vi "da Eq.vi"(0 "Plane Lat":dbl, 1 "Plane Lon":dbl, 2 "Plane Height (ft)":dbl, 3 "Plane Roll":dbl, 4 "Plane Pitch":dbl, 5 "Plane Heading":dbl, 6 "Displayed Image:Size:All Elements":cluster{"Width":u32, "Height":u32}, 7 "Last Mouse Position:All Elements":cluster{"X":i32, "Y":i32}) -> (16 "Latitude":dbl, 17 "Longitude":dbl)   [LabVIEW 2014]
panel:
  in  "Horizontal View Angle":dbl=74.0
  in  "Verticle View Angle":dbl=60.0
  # "AXIS 207MW has a horizontal view angle of 74 deg\nand a verticle view angle of 60 deg"
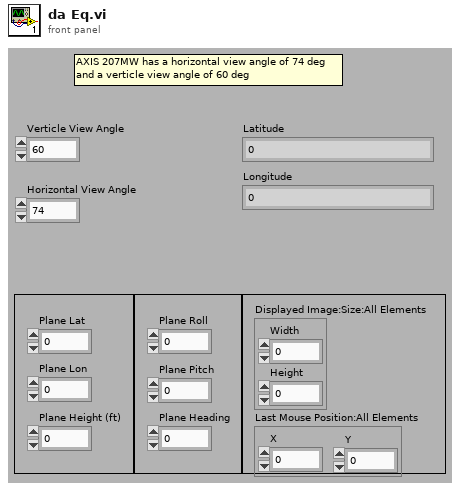
[diagram p1: front panel]
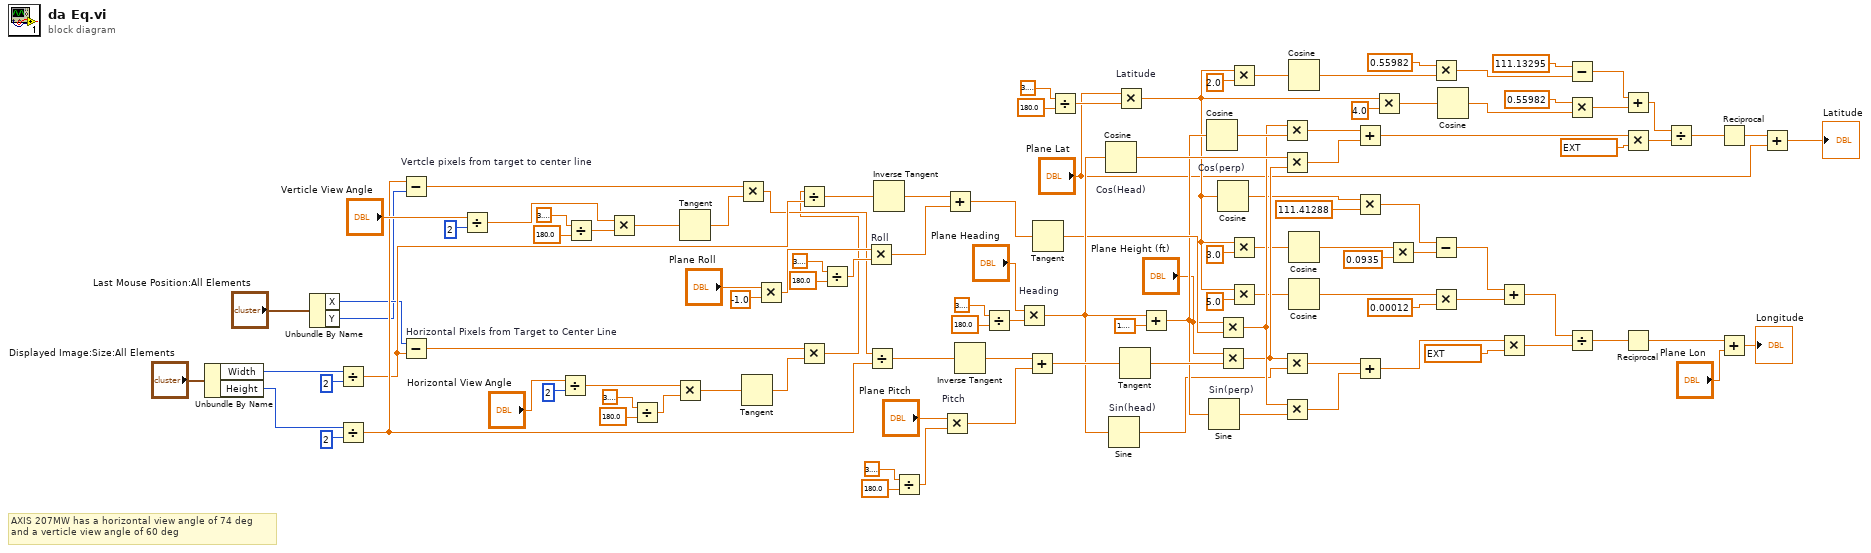
[diagram p0: block diagram]
diagram:
  # "AXIS 207MW has a horizontal view angle of 74 deg\nand a verticle view angle of 60 deg"
  n1 = Unbundle By Name("Displayed Image:Size:All Elements") -> ("Width"=w53:u32, "Height"=w52:u32)
  n2 = Unbundle By Name("Last Mouse Position:All Elements") -> ("X"=w4:i32, "Y"=w3:i32)
  n3 = Divide(x=w53, y=u32 2) -> (x/y=w82:dbl)
  n4 = Divide(x=w52, y=u32 2) -> (x/y=w108:dbl)
  n5 = Subtract "Vertcle pixels from target to center line"(x=w108, y=w3) -> (x-y=w109:dbl)
  n6 = Subtract "Horizontal Pixels from Target to Center Line"(x=w4, y=w82) -> (x-y=w91:dbl)
  n7 = Divide(x="Verticle View Angle", y=u32 2) -> (x/y=w107:dbl)
  n8 = Divide(x="Horizontal View Angle", y=u32 2) -> (x/y=w87:dbl)
  n9 = Divide(x=3.141592653589793, y=180.0) -> (x/y=w104:dbl)
  n10 = Multiply(x=w107, y=w104) -> (x*y=w103:dbl)
  n11 = Divide(x=3.141592653589793, y=180.0) -> (x/y=w90:dbl)
  n12 = Multiply(x=w87, y=w90) -> (x*y=w84:dbl)
  n13 = Tangent(1:w103) -> (0:w102:dbl)
  n14 = Multiply(x=w109, y=w102) -> (x*y=w2:dbl)
  n15 = Tangent(1:w84) -> (0:w83:dbl)
  n16 = Multiply(x="Plane Roll", y=-1.0) -> (x*y=w6:dbl)
  n17 = Multiply(x=w91, y=w83) -> (x*y=w1:dbl)
  n18 = Divide(x=w1, y=w82) -> (x/y=w81:dbl)
  n19 = Divide(x=3.141592653589793, y=180.0) -> (x/y=w77:dbl)
  n20 = Multiply "Roll"(x=w6, y=w77) -> (x*y=w76:dbl)
  n21 = Divide(x=w2, y=w108) -> (x/y=w101:dbl)
  n22 = Inverse Tangent(1:w81) -> (0:w80:dbl)
  n23 = Divide(x=3.141592653589793, y=180.0) -> (x/y=w99:dbl)
  n24 = Multiply "Pitch"(x="Plane Pitch", y=w99) -> (x*y=w96:dbl)
  n25 = Add(x=w80, y=w76) -> (x+y=w75:dbl)
  n26 = Inverse Tangent(1:w101) -> (0:w100:dbl)
  n27 = Divide(x=3.141592653589793, y=180.0) -> (x/y=w92:dbl)
  n28 = Multiply "Heading"(x="Plane Heading", y=w92) -> (x*y=w51:dbl)
  n29 = Add(x=w100, y=w96) -> (x+y=w95:dbl)
  n30 = Tangent(1:w75) -> (0:w50:dbl)
  n31 = Divide(x=3.141592653589793, y=180.0) -> (x/y=w66:dbl)
  n32 = Cosine "Cos(Head)"(x=w51) -> (cos(x)=w48:dbl)
  n33 = Sine "Sin(head)"(x=w51) -> (sin(x)=w41:dbl)
  n34 = Multiply "Latitude"(x="Plane Lat", y=w66) -> (x*y=w25:dbl)
  n35 = Tangent(1:w95) -> (0:w49:dbl)
  n36 = Add(x=w51, y=1.5707963267948966) -> (x+y=w47:dbl)
  n37 = Cosine "Cos(perp)"(x=w47) -> (cos(x)=w45:dbl)
  n38 = Sine "Sin(perp)"(x=w47) -> (sin(x)=w43:dbl)
  n39 = Cosine(x=w25) -> (cos(x)=w35:dbl)
  n40 = Multiply(x="Plane Height (ft)", y=w50) -> (x*y=w42:dbl)
  n41 = Multiply(x="Plane Height (ft)", y=w49) -> (x*y=w40:dbl)
  n42 = Multiply(x=w25, y=2.0) -> (x*y=w67:dbl)
  n43 = Multiply(x=w25, y=3.0) -> (x*y=w31:dbl)
  n44 = Multiply(x=w25, y=5.0) -> (x*y=w27:dbl)
  n45 = Multiply(x=w42, y=w45) -> (x*y=w44:dbl)
  n46 = Multiply(x=w48, y=w40) -> (x*y=w46:dbl)
  n47 = Multiply(x=w40, y=w41) -> (x*y=w39:dbl)
  n48 = Multiply(x=w42, y=w43) -> (x*y=w38:dbl)
  n49 = Cosine(x=w67) -> (cos(x)=w68:dbl)
  n50 = Cosine(x=w31) -> (cos(x)=w29:dbl)
  n51 = Cosine(x=w27) -> (cos(x)=w23:dbl)
  n52 = Add(x=w44, y=w46) -> (x+y=w73:dbl)
  n53 = Multiply(x=w35, y=111.41288) -> (x*y=w33:dbl)
  n54 = Add(x=w39, y=w38) -> (x+y=w37:dbl)
  n55 = Multiply(x=w25, y=4.0) -> (x*y=w62:dbl)
  n56 = Multiply(x=w29, y=0.0935) -> (x*y=w28:dbl)
  n57 = Multiply(x=0.55982, y=w68) -> (x*y=w70:dbl)
  n58 = Subtract(x=w33, y=w28) -> (x-y=w22:dbl)
  n59 = Multiply(x=w23, y=0.00012) -> (x*y=w21:dbl)
  n60 = Cosine(x=w62) -> (cos(x)=w61:dbl)
  n61 = Add(x=w22, y=w21) -> (x+y=w19:dbl)
  n62 = Multiply(x=w37, y=ext 0.0003048) -> (x*y=w20:ext)
  n63 = Subtract(x=111.13295, y=w70) -> (x-y=w59:dbl)
  n64 = Multiply(x=0.55982, y=w61) -> (x*y=w58:dbl)
  n65 = Divide(x=w19, y=w20) -> (x/y=w18:ext)
  n66 = Add(x=w59, y=w58) -> (x+y=w57:dbl)
  n67 = Multiply(x=w73, y=ext 0.0003048) -> (x*y=w56:ext)
  n68 = Reciprocal(x=w18) -> (1/x=w14:ext)
  n69 = Divide(x=w57, y=w56) -> (x/y=w55:ext)
  n70 = Reciprocal(x=w55) -> (1/x=w15:ext)
  n71 = Add(x=w14, y="Plane Lon") -> (x+y=→"Longitude":ext)
  n72 = Add(x=w15, y="Plane Lat") -> (x+y=→"Latitude":ext)
